vi "ComparaDataUART.vi"(8 "error in (no error)":errorcluster, 10 "StringIN":string, 11 "XuLyStringUART in":refnum<class "XuLyStringUART.lvclass">) -> (0 "error out":errorcluster, 3 "XuLyStringUART out":refnum<class "XuLyStringUART.lvclass">)   [LabVIEW 2014, in "LibraryGcode.lvlib" / "XuLyStringUART.lvclass"]
uses:
  XuLyStringUART.lvclass
  XuLyStringUART.lvclass/XuLyStringUART.ctl
  control/stateBoardFirmware.ctl
  LibraryGcode.lvlib
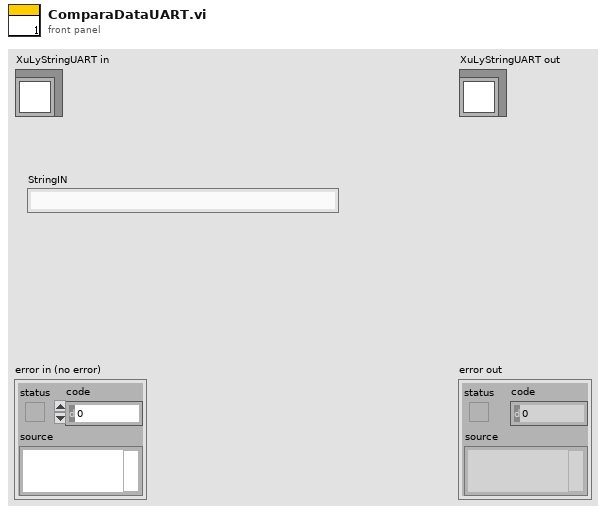
[diagram p1: front panel]
types:
  T1 = typedef "LibraryGcode.lvlib/stateBoardFirmware.ctl" = enum16{"Running", "Waiting", "Pos", "IDLE"}
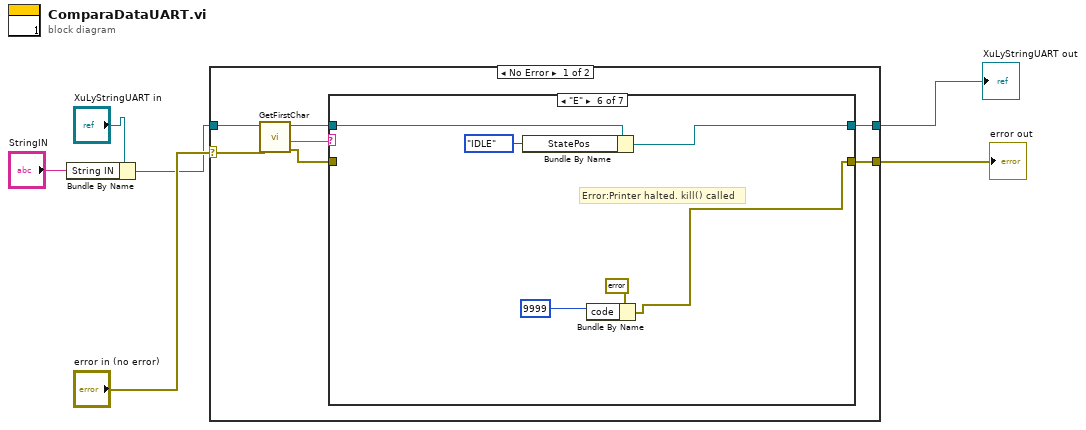
[diagram p0: block diagram]
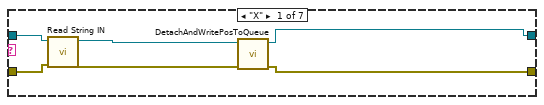
[diagram p2: hidden frame]
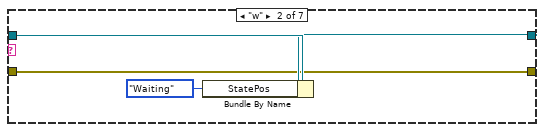
[diagram p3: hidden frame]
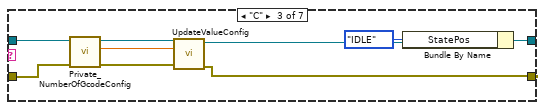
[diagram p4: hidden frame]
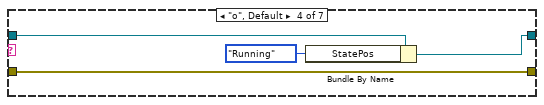
[diagram p5: hidden frame]
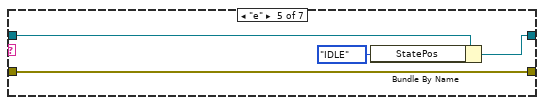
[diagram p6: hidden frame]
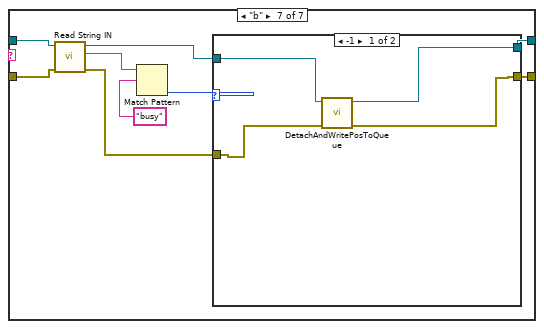
[diagram p7: hidden frame]
diagram:
  n1 = Bundle By Name(cluster="XuLyStringUART in", "String IN"="StringIN") -> (w3:refnum<class "XuLyStringUART.lvclass">)
  n2 = case shown="No Error" "error in (no error)" {
    selector: "error in (no error)" -> [w9 w63]
    tunnel: [w7 w63] -> w5
    tunnel: [w13 w62] -> w4
    tunnel: w3 -> [w12 w62]
    frame No Error {
      n3 = call-dynamic "GetFirstChar.vi"("error in (no error)"=w9, "XuLyStringUART in"=w12) -> ("error out"=w8:errorcluster, "First Char"=w10:string, "XuLyStringUART out"=w11:refnum<class "XuLyStringUART.lvclass">)  [unwired: 7 in]
      n4 = case shown="\"E\"" w10 {
        tunnel: w8 -> [w18 w20 w31 w36 w38 _ w51]
        tunnel: [w17 w20 w27 w36 w38 w41 w53] -> w7
        tunnel: [w16 w22 w25 w33 w37 w43 w47] -> w13
        tunnel: w11 -> [w19 w23 w32 w35 w40 w45 w52]
        frame "X" {
          n5 = call-dynamic "Read String IN.vi"("error in (no error)"=w18, "XuLyStringUART in"=w19) -> ("error out"=w14:errorcluster, "XuLyStringUART out"=w15:refnum<class "XuLyStringUART.lvclass">)  [unwired: 7 in, 1 out]
          n6 = call-dynamic "DetachAndWritePosToQueue.vi"("error in (no error)"=w14, "XuLyStringUART in"=w15) -> ("error out"=w17:errorcluster, "XuLyStringUART out"=w16:refnum<class "XuLyStringUART.lvclass">)  [unwired: 8 in]
        }
        frame "w" {
          n7 = Bundle By Name(cluster=w23, "StatePos"=stateBoardFirmware."Waiting" ("outPOS.StatePos")) -> (w22:refnum<class "XuLyStringUART.lvclass">)
        }
        frame "C" {
          n8 = call-dynamic "Private_NumberOfGcodeConfig.vi"("error in (no error)"=w31, "XuLyStringUART in"=w32) -> ("error out"=w28:errorcluster, "McodeConfigNumber"=w29:dbl, "XuLyStringUART out"=w30:refnum<class "XuLyStringUART.lvclass">)  [unwired: 7 in]
          n9 = call-dynamic "UpdateValueConfig.vi"("error in (no error)"=w28, "McodeConfigNumber"=w29, "XuLyStringUART in"=w30) -> ("error out"=w27:errorcluster, "XuLyStringUART out"=w26:refnum<class "XuLyStringUART.lvclass">)  [unwired: 7 in]
          n10 = Bundle By Name(cluster=w26, "StatePos"=stateBoardFirmware."IDLE" ("outPOS.StatePos")) -> (w25:refnum<class "XuLyStringUART.lvclass">)
        }
        frame "o", Default {
          n11 = Bundle By Name(cluster=w35, "StatePos"=stateBoardFirmware."Running" ("outPOS.StatePos")) -> (w33:refnum<class "XuLyStringUART.lvclass">)
        }
        frame "e" {
          n12 = Bundle By Name(cluster=w40, "StatePos"=stateBoardFirmware."IDLE" ("outPOS.StatePos")) -> (w37:refnum<class "XuLyStringUART.lvclass">)
        }
        frame "E" {
          # "Error:Printer halted. kill() called"
          n13 = Bundle By Name(cluster=w45, "StatePos"=stateBoardFirmware."IDLE" ("outPOS.StatePos")) -> (w43:refnum<class "XuLyStringUART.lvclass">)
          n14 = Bundle By Name(cluster=errorcluster {"status"=FALSE, "code"=0, "source"="REBOOT"} ("error IO"), "code"=9999) -> (w41:errorcluster)
        }
        frame "b" {
          n15 = call-dynamic "Read String IN.vi"("error in (no error)"=w51, "XuLyStringUART in"=w52) -> ("error out"=w49:errorcluster, "String IN"=w48:string, "XuLyStringUART out"=w50:refnum<class "XuLyStringUART.lvclass">)  [unwired: 7 in]
          n16 = Match Pattern(string=w48, regular expression="busy") -> (offset past match=w54:i32)  [unwired: 1 in, 3 out]
          n17 = case shown="-1" w54 {
            tunnel: w49 -> [w57 w60]
            tunnel: w50 -> [w59 w61]
            tunnel: [w58 w61] -> w47
            tunnel: [w56 w60] -> w53
            frame -1 {
              n18 = call-dynamic "DetachAndWritePosToQueue.vi"("error in (no error)"=w57, "XuLyStringUART in"=w59) -> ("error out"=w56:errorcluster, "XuLyStringUART out"=w58:refnum<class "XuLyStringUART.lvclass">)  [unwired: 8 in]
            }
            frame Default {
            }
          }
        }
      }
    }
    frame Error {
    }
  }
  "error out" <- w5
  "XuLyStringUART out" <- w4
